vi "Execute Control Visible Toggle(Multi-select).vi"(6 "Mouse Position":T1 caption="鼠标位置", 8 "User VI Ref":refnum<vi> caption="用户VI引用", 9 "Menu Item Tag Suffix":string caption="菜单项标签后缀", 10 "Remaining Items":refnum<vi>[](array[refnum]) caption="剩余项", 11 "Affected Items":T2 caption="受影响的项") -> (0 "Fail transaction?":bool caption="操作失败？")   [LabVIEW 2020]
doc: "该VI属于修改LabVIEW快捷菜单部分。这是用户选择快捷菜单时调用的执行VI。该VI执行选中菜单项的操作。"
uses:
  Control Visible Toggle.ctl
  <vilib>/Utility/miscctls.llb/LVPositionTypeDef.ctl
panel:
  # "除“受影响的项”之外，前面板上的其他所有控件都已锁定，以防被意外编辑。修改控件名称或类型，而不是“受影响的项”簇的元素将使VI无法作为菜单插件使用。\n\n请参考每个控件的即时帮助了解其用法。"
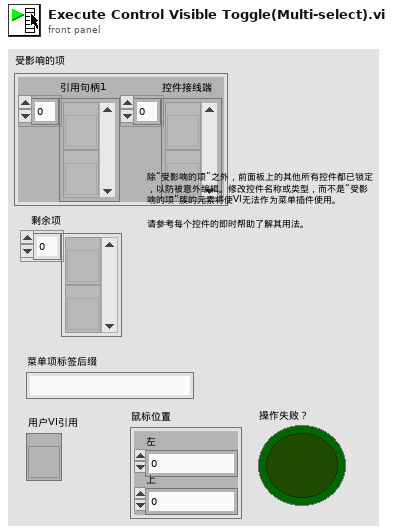
[diagram p1: front panel]
types:
  T1 = typedef "LVPositionTypeDef.ctl" = cluster{"Left":i32, "Top":i32}
  T2 = typedef "Control Visible Toggle.ctl" = cluster{"Control":refnum<vi>[], "Control Term":refnum<vi>[]}
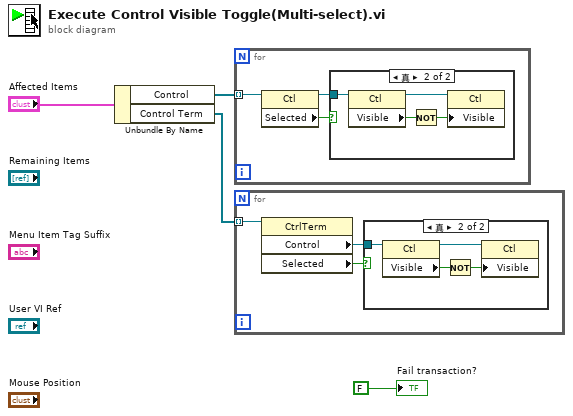
[diagram p0: block diagram]
diagram:
  n1 = Unbundle By Name("Affected Items") -> ("Control"=w2:refnum<vi>[], "Control Term"=w1:refnum<vi>[])
  n2 = for {
    tunnel: w2 -> [w7] mode=indexing
    n3 = property class="Ctl"(reference=w7) -> (reference out=w6:refnum<vi>, "Selected"=w5:bool)  [unwired: 1 in, 1 out]
    n4 = case shown="真" w5 {
      tunnel: w6 -> [_ w8]
      frame False {
      }
      frame True {
        n5 = property class="Ctl"(reference=w8) -> (reference out=w9:refnum<vi>, "Visible"=w10:bool)  [unwired: 1 in, 1 out]
        n6 = Not(x=w10) -> (.not. x?=w11:bool)
        n7 = property class="Ctl"(reference=w9, "Visible"=w11) -> ()  [unwired: 1 in, 2 out]
      }
    }
  }
  n8 = for {
    tunnel: w1 -> [w14] mode=indexing
    n9 = property class="CtrlTerm"(reference=w14) -> ("Control"=w12:refnum<vi>, "Selected"=w13:bool)  [unwired: 1 in, 2 out]
    n10 = case shown="真" w13 {
      tunnel: w12 -> [_ w15]
      frame False {
      }
      frame True {
        n11 = property class="Ctl"(reference=w15) -> (reference out=w16:refnum<vi>, "Visible"=w17:bool)  [unwired: 1 in, 1 out]
        n12 = Not(x=w17) -> (.not. x?=w18:bool)
        n13 = property class="Ctl"(reference=w16, "Visible"=w18) -> ()  [unwired: 1 in, 2 out]
      }
    }
  }
  "Fail transaction?" <- FALSE ("Fail transaction?")
